vi "PH_4_Pos_Selector.Picture PA Movable Lens.vi"(1 "Current Position":T1 items=["unknown", "Position I", "Position II", "Position III", "Position IV", "moving"]) -> (0 "Movable Lens Array":picture[](array[picture]))   [LabVIEW 2014, in "PH_4_Pos_Selector.lvlib"]
uses:
  PH_4_Pos_Selector.lvlib
  PH_4_Pos_Selector.Position Selector.ctl
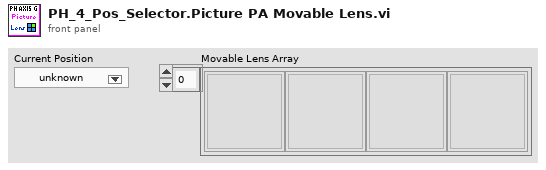
[diagram p1: front panel]
types:
  T1 = typedef "PH_4_Pos_Selector.lvlib/PH_4_Pos_Selector.Position Selector.ctl" = u16
  T2 = cluster{"left":i16, "top":i16, "right":i16, "bottom":i16}[]
  T3 = cluster{"left":i16, "top":i16, "right":i16, "bottom":i16}
  T4 = cluster{"horizontal":enum16{"left", "center", "right"}, "vertical":enum16{"top", "center", "bottom"}}
  T5 = enum16{"User-specified Font", "Application Font", "System Font", "Dialog Font"}
  T6 = cluster{"Font Name:":string, "Size":i16, "Strikeout?":bool, "Italic?":bool, "Underline?":bool, "Outline?":bool, "Shadow?":bool, "Bold?":bool}
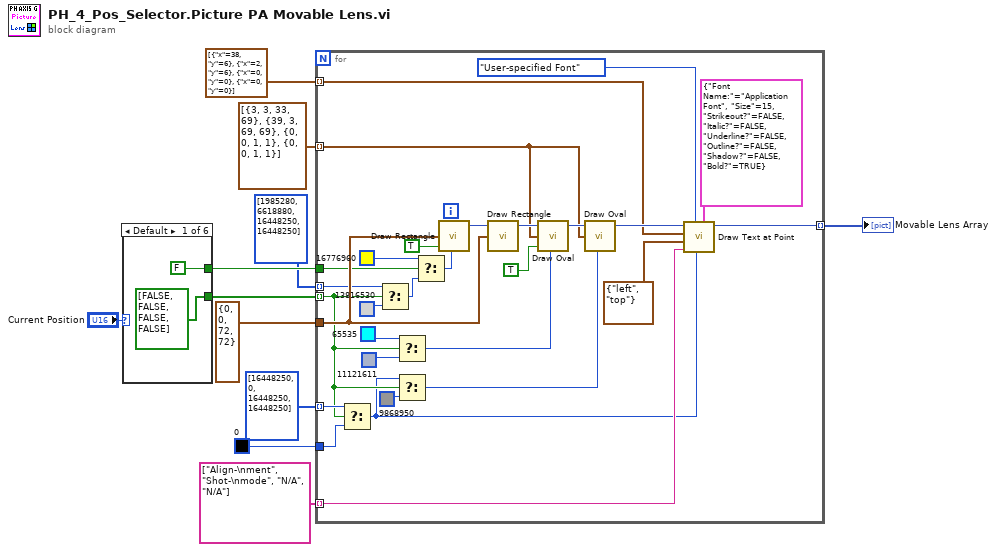
[diagram p0: block diagram]
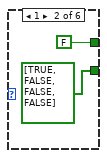
[diagram p2: hidden frame]
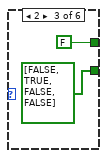
[diagram p3: hidden frame]
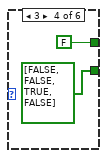
[diagram p4: hidden frame]
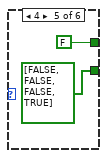
[diagram p5: hidden frame]
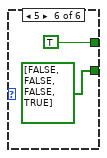
[diagram p6: hidden frame]
diagram:
  n1 = case shown="Default" "Current Position" {
    tunnel: [bool[] [FALSE, FALSE, FALSE, FALSE] bool[] [TRUE, FALSE, FALSE, FALSE] bool[] [FALSE, TRUE, FALSE, FALSE] bool[] [FALSE, FALSE, TRUE, FALSE] bool[] [FALSE, FALSE, FALSE, TRUE] bool[] [FALSE, FALSE, FALSE, TRUE]] -> w10
    tunnel: [FALSE FALSE FALSE FALSE FALSE TRUE] -> w9
    frame Default {
    }
    frame 1 {
    }
    frame 2 {
    }
    frame 3 {
    }
    frame 4 {
    }
    frame 5 {
    }
  }
  n2 = for {
    tunnel: T3 {"left"=0, "top"=0, "right"=72, "bottom"=72} ("rect") -> [w51]
    tunnel: w10 -> [w30] mode=indexing
    tunnel: w9 -> [w48]
    tunnel: [w42] -> w2 mode=indexing
    tunnel: string[] ["Align-\nment", "Shot-\nmode", "N/A", "N/A"] -> [w43] mode=indexing
    tunnel: u32[] [1985280, 6618880, 16448250, 16448250] -> [w41] mode=indexing
    tunnel: u32[] [16448250, 0, 16448250, 16448250] -> [w40] mode=indexing
    tunnel: u32 0 -> [w39]
    tunnel: cluster{"x":i16, "y":i16}[] [{"x"=38, "y"=6}, {"x"=2, "y"=6}, {"x"=0, "y"=0}, {"x"=0, "y"=0}] -> [w25] mode=indexing
    tunnel: T2 [{"left"=3, "top"=3, "right"=33, "bottom"=69}, {"left"=39, "top"=3, "right"=69, "bottom"=69}, {"left"=0, "top"=0, "right"=1, "bottom"=1}, {"left"=0, "top"=0, "right"=1, "bottom"=1}] -> [w26] mode=indexing
    n3 = Select(t=w40, s=w30, f=w39) -> (s? t:f=w29:u32)
    n4 = Select(t=w41, s=w30, f=u32 13816530) -> (s? t:f=w46:u32)
    n5 = Select(t=u32 65535 ("color(black)"), s=w30, f=u32 11121611) -> (s? t:f=w32:u32)
    n6 = Select(t=w29, s=w30, f=u32 9868950) -> (s? t:f=w28:u32)
    n7 = Select(t=u32 16776960, s=w48, f=w46) -> (s? t:f=w45:u32)
    n8 = call <vilib>:"Draw Rectangle.vi"("rect"=w51, "fill?(F)"=TRUE, "color(black)"=w45) -> ("new picture"=w52:picture)  [unwired: 6 in]
    n9 = call <vilib>:"Draw Rectangle.vi"("picture"=w52, "rect"=w51) -> ("new picture"=w37:picture)  [unwired: 7 in]
    n10 = call <vilib>:"Draw Oval.vi"("picture"=w37, "rect"=w26, "fill?(F)"=TRUE, "color(black)"=w32) -> ("new picture"=w36:picture)  [unwired: 5 in]
    n11 = call <vilib>:"Draw Oval.vi"("picture"=w36, "rect"=w26, "color(black)"=w28) -> ("new picture"=w35:picture)  [unwired: 6 in]
    n12 = call <vilib>:"Draw Text at Point.vi"("[user-specified font]"=T6 {"Font Name:"="Application Font", "Size"=15, "Strikeout?"=FALSE, "Italic?"=FALSE, "Underline?"=FALSE, "Outline?"=FALSE, "Shadow?"=FALSE, "Bold?"=TRUE}, "text color(black)"=w29, "desired font(Application)"=T5."User-specified Font", "text"=w43, "alignment(left, top)"=T4 {"horizontal"=enum."left", "vertical"=enum."top"}, "origin"=w25, "picture"=w35) -> ("new picture"=w42:picture)  [unwired: 3 in, 1 out]
  }
  "Movable Lens Array" <- w2
